vi "BRig_RT__Case_Exp__State_SelectPre__v2.vi"(0 "input_dataCurrent":u16[](array[numeric]), 1 "input_SelectWrong":bool, 2 "input_SelectReward":bool, 5 "input_dataExp":u16[](array[numeric]), 7 "input_LickL":bool, 9 "input_LickR":bool, 11 "input_arrTrig":bool[](array[boolean])) -> (3 "output_state":T1, 4 "output_dataCurrent":u16[](array[numeric]), 8 "output_l1_laserEvent":bool, 10 "output_l1_laserOn":bool, 13 "output_l2_laserOn":bool, 14 "output_l2_laserEvent":bool)   [LabVIEW 2014]
uses:
  myRIO_BRig_RT__Case_Exp_stateList.ctl
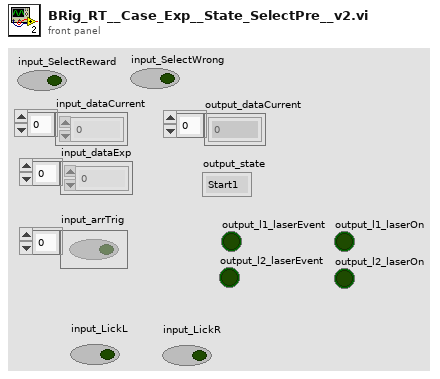
[diagram p1: front panel]
types:
  T1 = typedef "myRIO_BRig_RT__Case_Exp_stateList.ctl" = enum16{"Start1", "Start2", "Start3", "saveSettings1", "saveSettings2", "saveSettings3", "saveSettings4", "saveSettings_LC_ENL_l1", "saveSettings_LC_ENL_l2", "saveSettings_LC_Cue_l1", "saveSettings_LC_Cue_l2", "saveSettings6_LC_l1_Other", "SaveSettings6_LC_l2_Other", "setSettings_Audio", "setSettings_Laser", "initBlock_pre", "initBlock", "initBlock2", "initBlock_post", "initTrial_pre", "initTrial", "initTrial2", "initTrial3", "initTrial4", "initTrial_LC_ENL1", "initTrial_LC_Cue1", "initTrial_LC_Cue1_2", "initTrial_LC_Sel", "initTrial_post", "ENL1_pre", "ENL1", "ENL1_post", "ENL1Penalty_pre", "ENL1Penalty", "ENL2_pre", "ENL2", "ENL2Penalty_pre", "ENL2Penalty", "Cue1_pre", "Cue1", "Cue1_post", "Cue1Penalty_pre", "Cue1Penalty", "Cue2_pre", "Cue2", "Cue2Penalty_pre", "Cue2Penalty", "Selection_pre", "Selection", "Select_post", "SelectReward_pre", "SelectReward", "SelectRewardPost_pre", "SelectRewardPost", "SelectWrong_pre", "SelectWrong", "SelectWrong_post", "SelectTimeout_pre", "SelectTimeout", "SelectTimeout_post", "endTrial_pre", "endTrial1", "endTrial2", "endTrial3", "endTrial_post", "endBlock_pre", "endBlock", "endBlock_post", "endExp", "commConnect", "commUpload_pre", "commUpload_dataBlock", "commUpload_dataCurrent", "commUpload_dataExp", "commUpload_dataLC", "commUpload_dataTrial", "commUpload_post", "saveData_pre", "saveData_dataBlock", "saveData_dataCurrent", "saveData_dataExp", "saveData_dataLC", "saveData_dataTrial", "saveData_post", "empty_endBlock1", "empty_endBlock2", "empty_endTrial1", "empty_endTrial2", "empty_endTrial3", "empty_endTrial4", "empty_endTrial5", "dummyState", "dummyState_endBlock", "FreeReward_pre", "FreeReward", "FreeRewardPost_pre", "FreeRewardPost"}
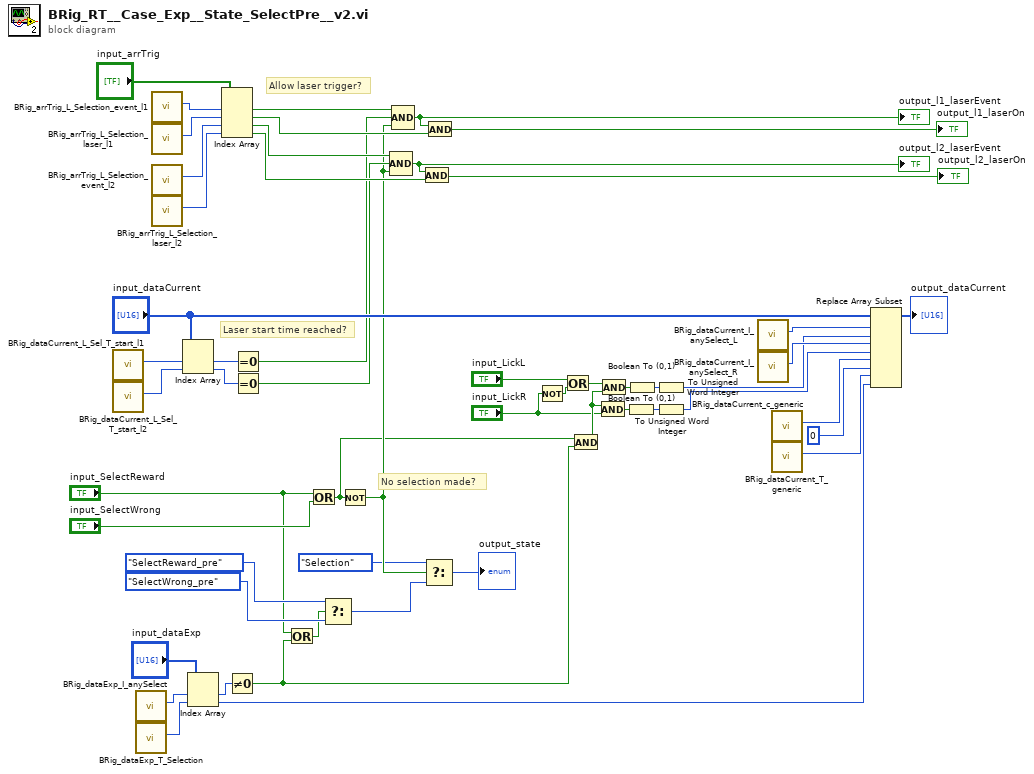
[diagram p0: block diagram]
diagram:
  # "No selection made?"
  # "Laser start time reached?"
  # "Allow laser trigger?"
  n1 = call "BRig_dataCurrent_L_Sel_T_start_l1.vi"() -> ("output_L_Sel_T_start_l1"=w41:i32)  [unwired: 11 in]
  n2 = call "BRig_dataCurrent_L_Sel_T_start_l2.vi"() -> ("output_L_Sel_T_start_l2"=w42:i32)  [unwired: 11 in]
  n3 = call "BRig_dataExp_I_anySelect.vi"() -> ("output_I_anySelect"=w38:i32)  [unwired: 11 in]
  n4 = call "BRig_dataExp_T_Selection.vi"() -> ("output_T_Selection"=w39:i32)  [unwired: 11 in]
  n5 = call "BRig_arrTrig_L_Selection_event_l1.vi"() -> ("output_L_Sel_event_l1"=w25:i32)  [unwired: 11 in]
  n6 = call "BRig_arrTrig_L_Selection_laser_l1.vi"() -> ("output_L_Sel_laserTrig_l1"=w24:i32)  [unwired: 11 in]
  n7 = call "BRig_arrTrig_L_Selection_event_l2.vi"() -> ("output_L_Sel_event_l2"=w23:i32)  [unwired: 11 in]
  n8 = call "BRig_arrTrig_L_Selection_laser_l2.vi"() -> ("output_L_Sel_laserTrig_l2"=w22:i32)  [unwired: 11 in]
  n9 = Index Array(array="input_dataCurrent", index #1=w41, index #2=w42) -> (element #1=w49:u16, element #2=w48:u16)
  n10 = Index Array(array="input_dataExp", index #1=w38, index #2=w39) -> (element #1=w37:u16, element #2=w1:u16)
  n11 = Index Array(array="input_arrTrig", index #1=w25, index #2=w24, index #3=w23, index #4=w22) -> (element #1=w14:bool, element #2=w18:bool, element #3=w15:bool, element #4=w20:bool)
  n12 = Not Equal To 0?(x=w37) -> (x != 0?=w4:bool)
  n13 = Equal To 0?(x=w49) -> (x = 0?=w13:bool)
  n14 = Equal To 0?(x=w48) -> (x = 0?=w12:bool)
  n15 = Or(x="input_SelectReward", y=w4) -> (x .or. y?=w7:bool)
  n16 = Or(x="input_SelectReward", y="input_SelectWrong") -> (x .or. y?=w5:bool)
  n17 = Select(t=myRIO_BRig_RT__Case_Exp_stateList."SelectReward_pre" ("Enum"), s=w7, f=myRIO_BRig_RT__Case_Exp_stateList."SelectWrong_pre" ("Enum")) -> (s? t:f=w11:T1)
  n18 = Not(x=w5) -> (.not. x?=w10:bool)
  n19 = Compound Arithmetic op=AND(w15, w12, w10) -> (w21:bool)
  "output_l2_laserEvent" <- w21
  n20 = Compound Arithmetic op=AND(w14, w13, w10) -> (w19:bool)
  "output_l1_laserEvent" <- w19
  n21 = And(x=w21, y=w20) -> (x .and. y?=→"output_l2_laserOn":bool)
  n22 = Select(t=myRIO_BRig_RT__Case_Exp_stateList."Selection" ("Enum"), s=w10, f=w11) -> (s? t:f=→"output_state":T1)
  n23 = And(x=w19, y=w18) -> (x .and. y?=→"output_l1_laserOn":bool)
  n24 = Not(x="input_LickR") -> (.not. x?=w27:bool)
  n25 = Or(x="input_LickL", y=w27) -> (x .or. y?=w26:bool)
  n26 = And(x=w5, y=w4) -> (x .and. y?=w34:bool)
  n27 = And(x=w34, y="input_LickR") -> (x .and. y?=w32:bool)
  n28 = And(x=w26, y=w34) -> (x .and. y?=w33:bool)
  n29 = Boolean To (0,1)(Boolean=w32) -> (0, 1=w30:i16)
  n30 = Boolean To (0,1)(Boolean=w33) -> (0, 1=w31:i16)
  n31 = To Unsigned Word Integer(number=w31) -> (unsigned 16bit integer=w3:u16)
  n32 = To Unsigned Word Integer(number=w30) -> (unsigned 16bit integer=w2:u16)
  n33 = call "BRig_dataCurrent_I_anySelect_L.vi"() -> ("output_IanySelect_L"=w36:i32)  [unwired: 11 in]
  n34 = call "BRig_dataCurrent_I_anySelect_R.vi"() -> ("output_IanySelect_R"=w35:i32)  [unwired: 11 in]
  n35 = call "BRig_dataCurrent_c_generic.vi"() -> ("output_count_generic"=w52:i32)  [unwired: 11 in]
  n36 = call "BRig_dataCurrent_T_generic.vi"() -> ("output_T_generic"=w51:i32)  [unwired: 11 in]
  n37 = Replace Array Subset(array="input_dataCurrent", new element #1=w3, index #1=w36, new element #2=w2, index #2=w35, new element #3=u16 0 ("new element/subarray"), index #3=w52, new element #4=w1, index #4=w51) -> (→"output_dataCurrent":u16[])
